vi "Read Credentials from File.vi"(8 "error in (no error)":errorcluster, 10 "path to aws credentials":path, 11 "Data.S3":refnum<class "Data.S3.lvclass">) -> (0 "error out":errorcluster, 3 "Data.S3 out":refnum<class "Data.S3.lvclass">)   [LabVIEW 2020, in "Data.S3.lvclass"]
uses:
  Data.S3.lvclass
  <vilib>/AWS Toolkit/Core/HTTP Request/AWS Credentials.ctl
  Data.S3.lvclass/Data.S3.ctl
  <vilib>/AWS Toolkit/Core/HTTP Request/HTTP Request.lvclass
panel:
  # "takes same credentials file as cli described here:\nhttps://docs.aws.amazon.com/cli/latest/userguide/cli-configure-files.html"
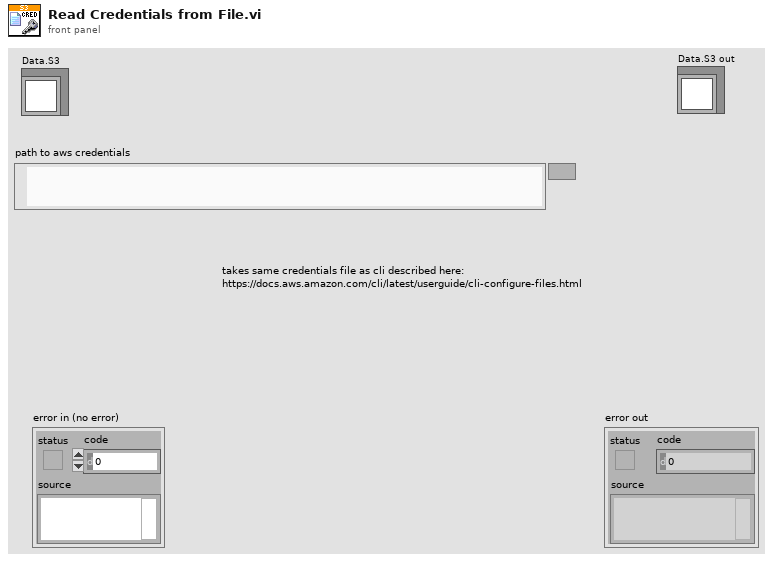
[diagram p1: front panel]
types:
  T1 = typedef "NI_AWS_Core.lvlib/HTTP Request.lvclass/AWS Credentials.ctl" = cluster{"Access Key":string, "Secret Key":string}
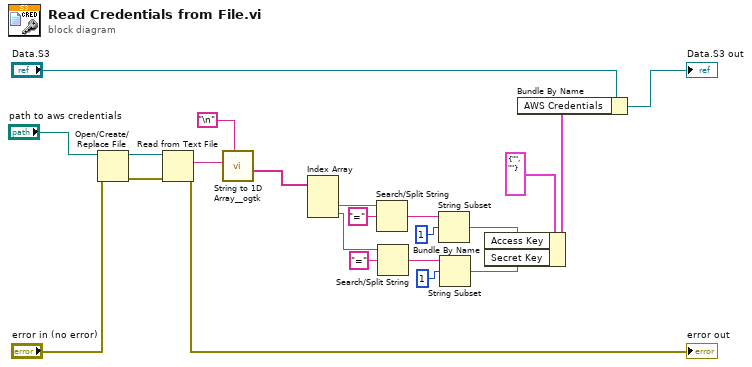
[diagram p0: block diagram]
diagram:
  n1 = Open/Create/Replace File(file path (use dialog)="path to aws credentials", error in="error in (no error)") -> (refnum out=w20:refnum<file>, error out=w19:errorcluster)  [unwired: 4 in, 1 out]
  n2 = Read from Text File(file (use dialog)=w20, error in=w19) -> (text=w17:string, error out=→"error out":errorcluster)  [unwired: 2 in, 2 out]
  n3 = call <userlib>:"String to 1D Array__ogtk.vi"("delimiter (Tab)"="\n", "string"=w17) -> ("Array of Strings"=w12:string[])  [unwired: 9 in]
  n4 = Index Array(array=w12) -> (element #2=w10:string, element #3=w3:string)  [unwired: 3 in, 1 out]
  n5 = Search/Split String(string=w10, search string/char (-)="=") -> (match + rest of string=w8:string)  [unwired: 1 in, 2 out]
  n6 = Search/Split String(string=w3, search string/char (-)="=") -> (match + rest of string=w5:string)  [unwired: 1 in, 2 out]
  n7 = String Subset(string=w8, offset (0)=1) -> (substring=w2:string)  [unwired: 1 in]
  n8 = String Subset(string=w5, offset (0)=1) -> (substring=w1:string)  [unwired: 1 in]
  n9 = Bundle By Name(cluster=T1 {"Access Key"="", "Secret Key"=""} ("AWS Credentials"), "Access Key"=w2, "Secret Key"=w1) -> (w13:T1)
  n10 = Bundle By Name(cluster="Data.S3", "AWS Credentials"=w13) -> (→"Data.S3 out":refnum<class "Data.S3.lvclass">)
